vi "SetTest.vi"(0 "reference in":refnum<class "MES_Local.lvclass">, 5 "Value":variant, 11 "error in (no error)":errorcluster) -> (4 "reference in":refnum<class "MES_Local.lvclass">, 6 "Cluster 2":T1={"Code"="", "Name"="", "Description"="", "Group"="", "IsGroup"=FALSE, "Tag"="", "Method"="", "Parrameter"="", "DataType"=enum."String", "Value"=variant, "Status"=enum."Pass", "LimitLo"=variant, "LimitHi"=variant, "StringMatch"="", "BooleanMatch"=FALSE, "DisplayFormat"="", "Units"="", "TestTime"=0.0}, 8 "Complete":bool, 10 "Pass":bool, 15 "error out":errorcluster)   [LabVIEW 2022 SP3, in "MES_Local.lvlib" / "MES_Local.lvclass"]
uses:
  MES_Local.lvclass
  Components/MES_Base.lvlibp/Controls/Test.ctl
  Components/MES_Base.lvlibp/Controls/Status.ctl
  <userlib>/_OpenG.lib/string/string.llb/Trim Whitespace (String)__ogtk.vi
  <vilib>/regexp/Match Regular Expression.xnode
  Components/MES_Base.lvlibp/MES_Base.lvclass
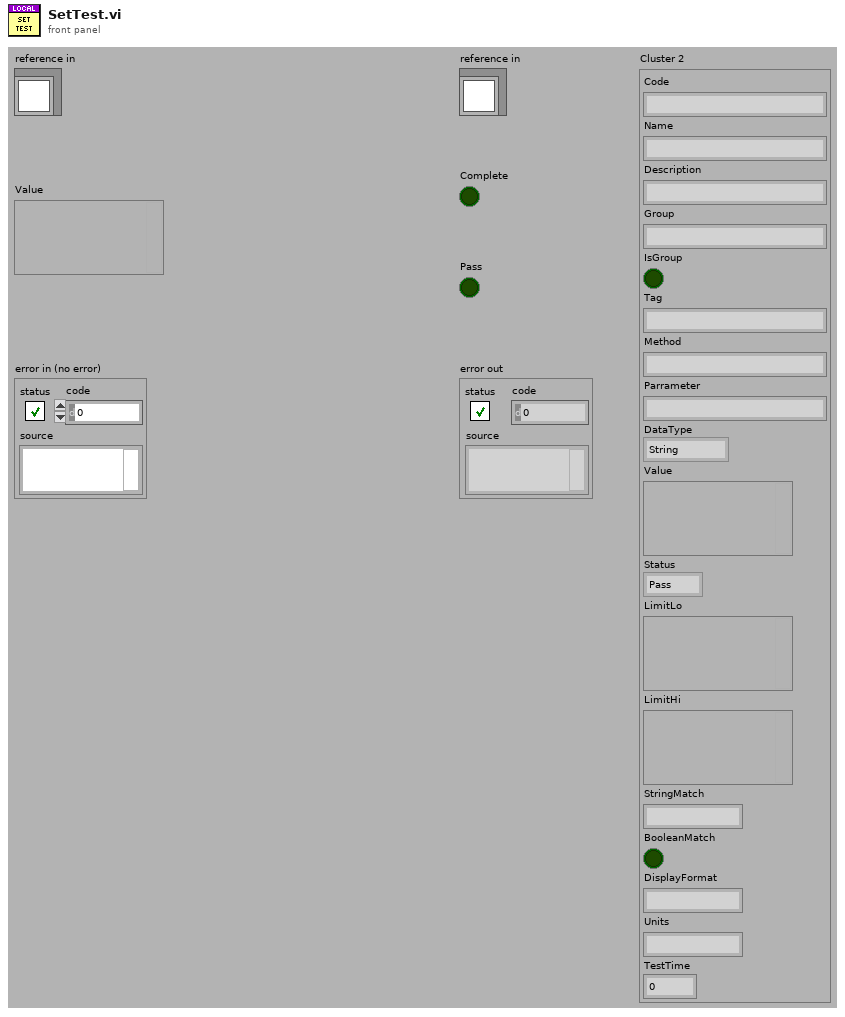
[diagram p1: front panel]
types:
  T1 = typedef "MES_Base.lvlibp/MES_Base.lvclass/Test.ctl" = cluster{"Code":string, "Name":string, "Description":string, "Group":string, "IsGroup":bool, "Tag":string, "Method":string, "Parrameter":string, "DataType":enum16{"NA", "String", "Boolean", "Int", "Dbl"}, "Value":variant, "Status":enum16{"Pending", "Pass", "Fail"}, "LimitLo":variant, "LimitHi":variant, "StringMatch":string, "BooleanMatch":bool, "DisplayFormat":string, "Units":string, "TestTime":dbl}
  T2 = typedef "MES_Base.lvlibp/MES_Base.lvclass/Status.ctl" = enum16{"Pending", "Pass", "Fail"}
  T3 = typedef "MES_Local.lvlib/MES_Local.lvclass/ObjectAttributes.ctl" = cluster{"Config":T4, "Logged_In?":bool, "AttributeNames":string[], "AttributeWritten":bool[], "ComponentNames":string[], "TestIndex":i32, "TestTag":string[], "Time Stamp":timestamp, "Employee":string, "Resource_Key":string, "Local Spec":path, "Login":refnum<class "Login_Base.lvclass">, "ReportPath":path, "Spec":T5, "StartTime":timestamp, "Role":string}
  T4 = typedef "MES_Local.lvlib/MES_Local.lvclass/Config.ctl" = cluster{"Results_Path":path}
  T5 = typedef "MES_Base.lvlibp/MES_Base.lvclass/Spec.ctl" = cluster{"Header":cluster{"Doctype":string, "Checksum":string, "DriverKey":string, "SpecId":string, "TransactionId":string, "AccountId":string, "SpecName":string, "WorkflowStep":string, "SerialNumber":string, "BatchNumber":string, "Status":enum16{"Pending", "Pass", "Fail"}, "Comment":string, "FirstFail":string, "Employee":string, "LocalMachine":string, "ResourceKey":string, "Date":string, "Time":string, "Duration":string, "DUT Position":i32}, "Components":cluster{"SerialNumber":string, "PartNumber":string, "Revision":string, "BatchNumber":string, "Name":string, "Description":string, "Attached":bool}[], "Attributes":cluster{"Name":string, "Description":string, "DataType":enum16{"NA", "String", "Boolean", "Int", "Dbl"}, "Value":variant, "DisplayFormat":string, "ReadOnly":bool, "Required":bool}[], "Tests":cluster{"Code":string, "Name":string, "Description":string, "Group":string, "IsGroup":bool, "Tag":string, "Method":string, "Parrameter":string, "DataType":enum16{"NA", "String", "Boolean", "Int", "Dbl"}, "Value":variant, "Status":enum16{"Pending", "Pass", "Fail"}, "LimitLo":variant, "LimitHi":variant, "StringMatch":string, "BooleanMatch":bool, "DisplayFormat":string, "Units":string, "TestTime":dbl}[]}
  T6 = cluster{"Code":string, "Name":string, "Description":string, "Group":string, "IsGroup":bool, "Tag":string, "Method":string, "Parrameter":string, "DataType":enum16{"NA", "String", "Boolean", "Int", "Dbl"}, "Value":variant, "Status":enum16{"Pending", "Pass", "Fail"}, "LimitLo":variant, "LimitHi":variant, "StringMatch":string, "BooleanMatch":bool, "DisplayFormat":string, "Units":string, "TestTime":dbl}[]
  T7 = cluster{"Code":string, "Name":string, "Description":string, "Group":string, "IsGroup":bool, "Tag":string, "Method":string, "Parrameter":string, "DataType":enum16{"NA", "String", "Boolean", "Int", "Dbl"}, "Value":variant, "Status":enum16{"Pending", "Pass", "Fail"}, "LimitLo":variant, "LimitHi":variant, "StringMatch":string, "BooleanMatch":bool, "DisplayFormat":string, "Units":string, "TestTime":dbl}
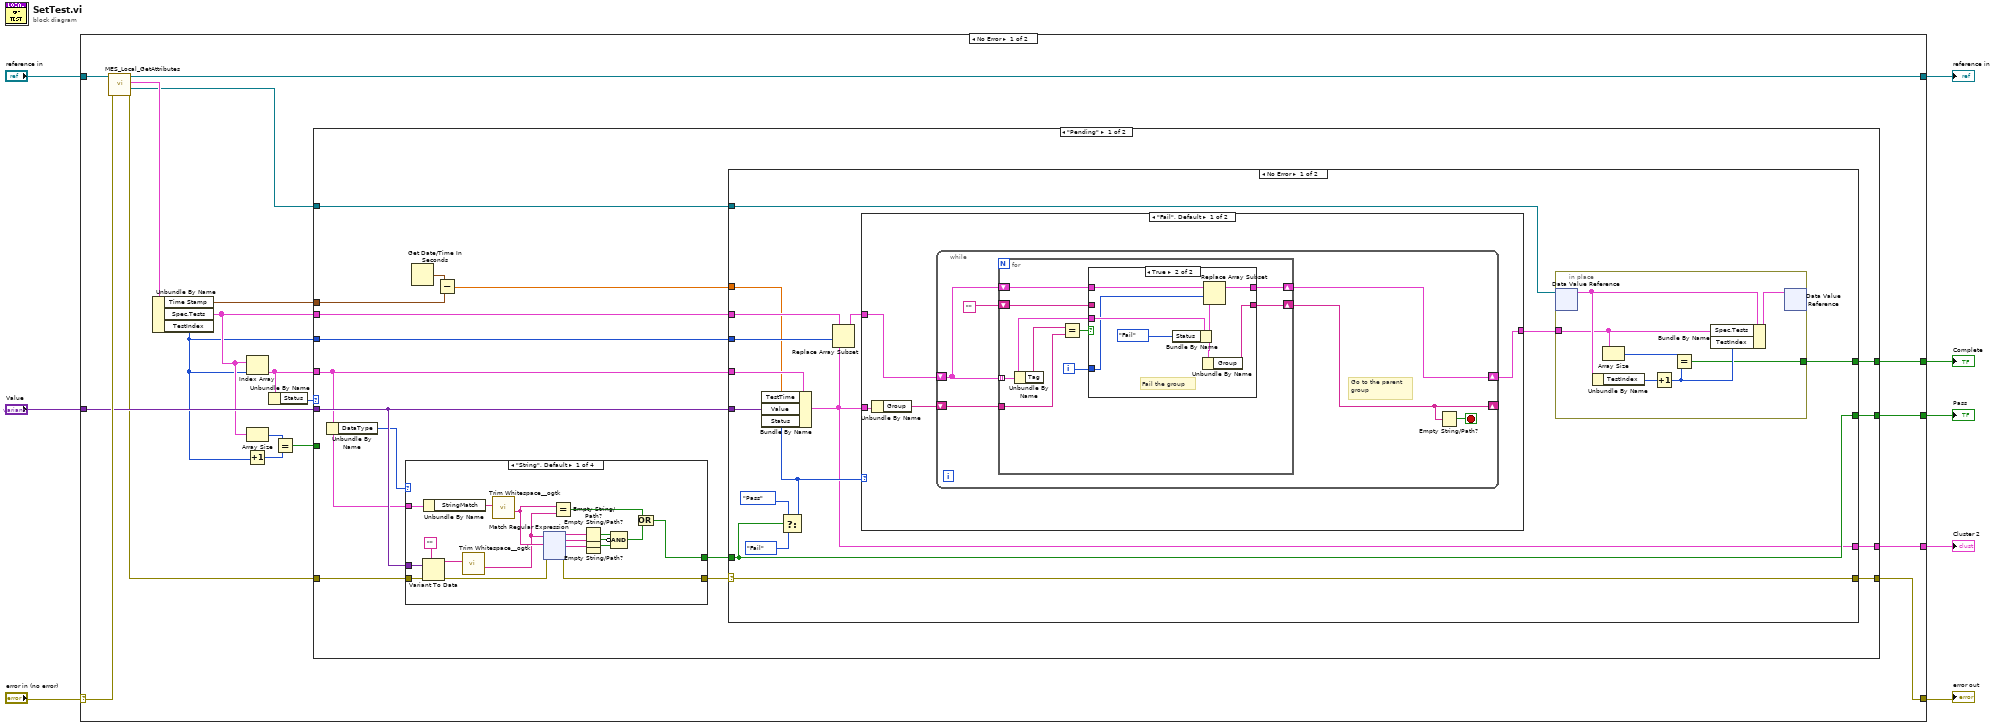
[diagram p0: block diagram]
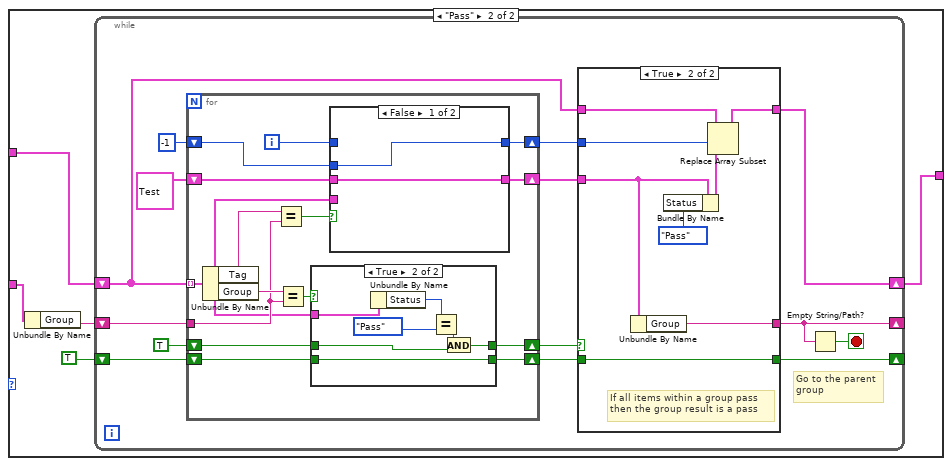
[diagram p3: hidden frame]
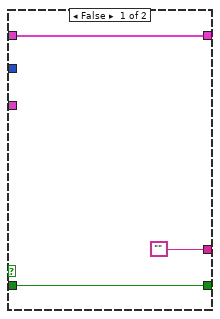
[diagram p4: hidden frame]
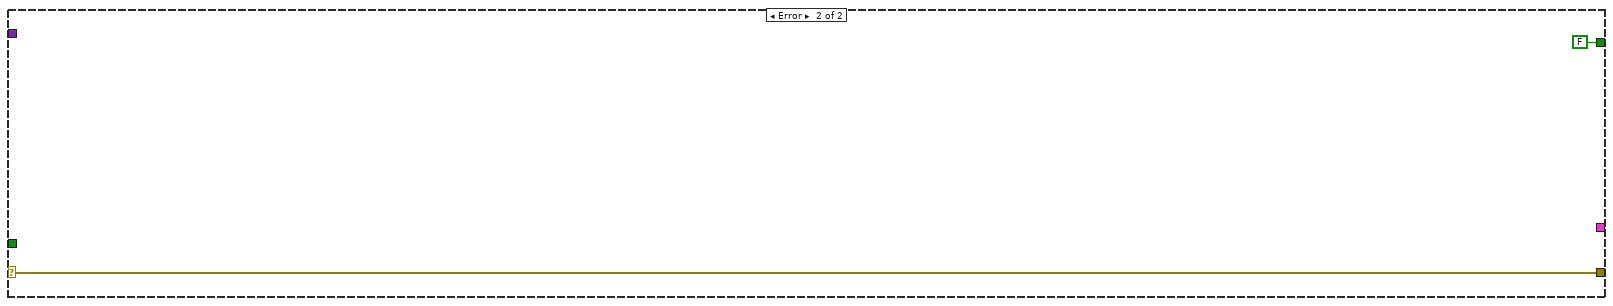
[diagram p7: hidden frame]
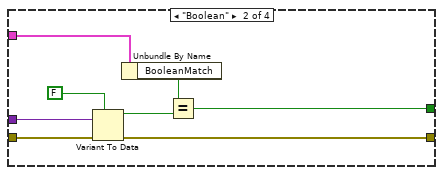
[diagram p8: hidden frame]
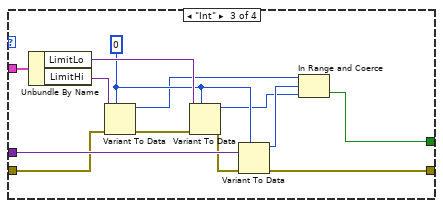
[diagram p9: hidden frame]
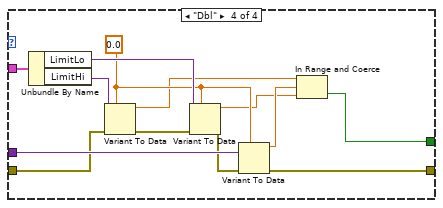
[diagram p10: hidden frame]
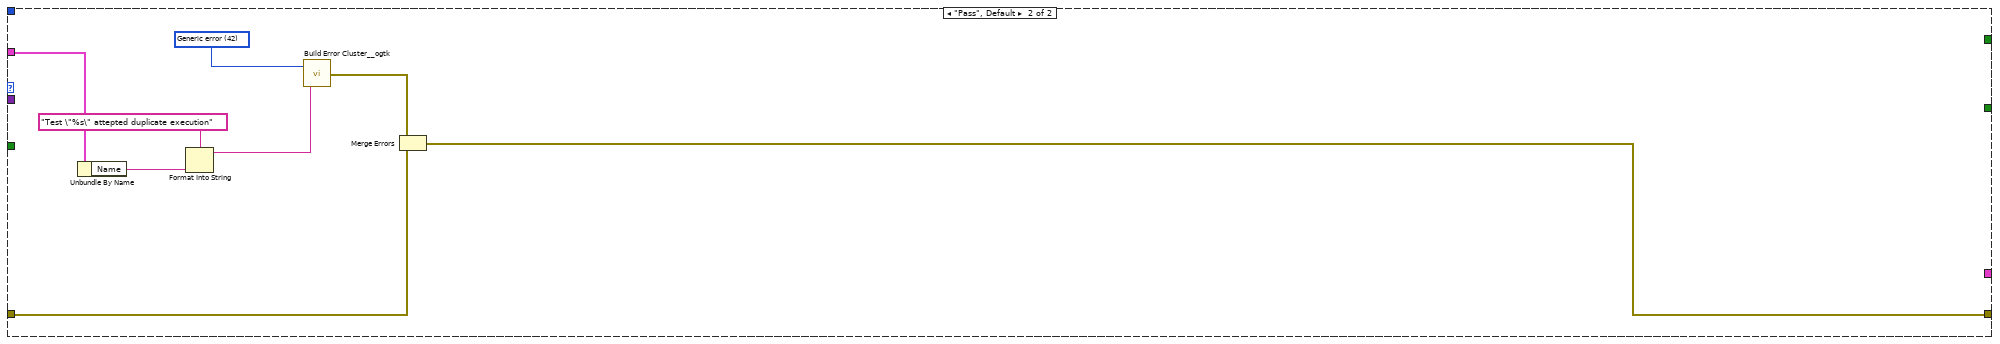
[diagram p11: hidden frame]
diagram:
  n1 = case shown="No Error" "error in (no error)" {
    selector: "error in (no error)" -> [w27 w333]
    tunnel: [w12 w333] -> w7
    tunnel: [w24 w332] -> w5
    tunnel: "reference in" -> [w25 w332]
    tunnel: "Value" -> [w19 _]
    tunnel: [w11 _] -> w3
    tunnel: [w10 _] -> w2
    tunnel: [w9 _] -> w1
    frame No Error {
      n2 = call "MES_Local_GetAttributes.vi"("error in (no error)"=w27, "reference in"=w25) -> ("error out"=w13:errorcluster, "DataRef"=w18:refnum<data-value>, "Data"=w26:T3, "reference out"=w24:refnum<class "MES_Local.lvclass">)  [unwired: 6 in]
      n3 = Unbundle By Name(w26) -> ("Time Stamp"=w17:timestamp, "Spec.Tests"=w16:T6, "TestIndex"=w15:i32)
      n4 = Index Array(array=w16, index=w15) -> (element=w23:T7)
      n5 = Increment(x=w15) -> (x+1=w20:i32)
      n6 = Array Size(array=w16) -> (size(s)=w21:i32)
      n7 = Unbundle By Name(w23) -> ("Status"=w22:enum16{"Pending", "Pass", "Fail"})
      n8 = Equal?(x=w21, y=w20) -> (x = y?=w14:bool)
      n9 = case shown="\"Pending\"" w22 {
        tunnel: w19 -> [w43 _]
        tunnel: w13 -> [w42 w329]
        tunnel: w18 -> [w41 _]
        tunnel: w16 -> [w38 _]
        tunnel: w15 -> [w37 _]
        tunnel: [w35 w328] -> w12
        tunnel: w17 -> [w33 _]
        tunnel: w23 -> [w31 w327]
        tunnel: [w30 _] -> w10
        tunnel: [w29 _] -> w9
        tunnel: [w28 _] -> w11
        tunnel: w14 -> [_ _]
        frame "Pending" {
          n10 = Unbundle By Name(w31) -> ("DataType"=w40:enum16{"NA", "String", "Boolean", "Int", "Dbl"})
          n11 = case shown="\"String\", Default" w40 {
            tunnel: w43 -> [w171 w296 w310 w323]
            tunnel: w42 -> [w172 w295 w306 w319]
            tunnel: [w161 w294 w309 w322] -> w36
            tunnel: w31 -> [w169 w293 w308 w321]
            tunnel: [w154 w290 w298 w311] -> w39
            frame "String", Default {
              n12 = Variant To Data(error in=w172, type="", Variant=w171) -> (data=w160:string, error out=w162:errorcluster)
              n13 = Unbundle By Name(w169) -> ("StringMatch"=w159:string)
              n14 = call-poly <userlib>:"Trim Whitespace__ogtk.vi"("String in"=w160) -> ("String out"=w157:string)  [unwired: 6 in]
              n15 = call-poly <userlib>:"Trim Whitespace__ogtk.vi"("String in"=w159) -> ("String out"=w158:string)  [unwired: 6 in]
              n16 = xnode "Match Regular Expression"("input string"=w157, "regular expression"=w158, "error in"=w162) -> ("before match"=w168:string, "whole match"=w165:string, "after match"=w164:string, "error out"=w161:errorcluster)  [unwired: 3 in, 1 out]
              n17 = Equal?(x=w158, y=w157) -> (x = y?=w156:bool)
              n18 = Empty String/Path?(string/path=w168) -> (empty?=w167:bool)
              n19 = Empty String/Path?(string/path=w165) -> (empty?=w166:bool)
              n20 = Empty String/Path?(string/path=w164) -> (empty?=w163:bool)
              n21 = Compound Arithmetic op=AND(w167, invert w166, w163) -> (w155:bool)
              n22 = Or(x=w156, y=w155) -> (x .or. y?=w154:bool)
            }
            frame "Boolean" {
              n23 = Variant To Data(error in=w295, type=FALSE, Variant=w296) -> (data=w292:bool, error out=w294:errorcluster)
              n24 = Unbundle By Name(w293) -> ("BooleanMatch"=w291:bool)
              n25 = Equal?(x=w291, y=w292) -> (x = y?=w290:bool)
            }
            frame "Int" {
              w302 = 0
              n26 = Unbundle By Name(w308) -> ("LimitLo"=w303:variant, "LimitHi"=w307:variant)
              n27 = Variant To Data(error in=w306, type=w302, Variant=w307) -> (data=w299:i32, error out=w305:errorcluster)
              n28 = Variant To Data(error in=w305, type=w302, Variant=w303) -> (data=w300:i32, error out=w304:errorcluster)
              n29 = Variant To Data(error in=w304, type=w302, Variant=w310) -> (data=w301:i32, error out=w309:errorcluster)
              n30 = In Range and Coerce(upper limit=w299, x=w301, lower limit=w300) -> (In Range?=w298:bool)  [unwired: 1 out]
            }
            frame "Dbl" {
              w315 = 0.0
              n31 = Unbundle By Name(w321) -> ("LimitLo"=w316:variant, "LimitHi"=w320:variant)
              n32 = Variant To Data(error in=w319, type=w315, Variant=w320) -> (data=w312:dbl, error out=w318:errorcluster)
              n33 = Variant To Data(error in=w318, type=w315, Variant=w316) -> (data=w313:dbl, error out=w317:errorcluster)
              n34 = Variant To Data(error in=w317, type=w315, Variant=w323) -> (data=w314:dbl, error out=w322:errorcluster)
              n35 = In Range and Coerce(upper limit=w312, x=w314, lower limit=w313) -> (In Range?=w311:bool)  [unwired: 1 out]
            }
          }
          n36 = Get Date/Time In Seconds() -> (seconds since 1Jan1904=w34:timestamp)
          n37 = Subtract(x=w34, y=w33) -> (x-y=w32:dbl)
          n38 = case shown="No Error" w36 {
            selector: w36 -> [w53 w153]
            tunnel: w43 -> [w58 _]
            tunnel: w41 -> [w57 _]
            tunnel: w31 -> [w56 _]
            tunnel: w39 -> [w47 _]
            tunnel: w38 -> [w51 _]
            tunnel: w37 -> [w52 _]
            tunnel: [w53 w153] -> w35
            tunnel: w32 -> [w49 _]
            tunnel: [w48 _] -> w30
            tunnel: [w47 FALSE] -> w29
            tunnel: [w46 _] -> w28
            frame No Error {
              n39 = Select(t=Status."Pass" ("Status"), s=w47, f=Status."Fail" ("Status")) -> (s? t:f=w55:T2)
              n40 = Bundle By Name(cluster=w56, "TestTime"=w49, "Value"=w58, "Status"=w55) -> (w46:T7)
              n41 = Replace Array Subset(array=w51, new element=w46, index=w52) -> (w50:T6)
              n42 = case shown="\"Fail\", Default" w55 {
                tunnel: w46 -> [w61 w91]
                tunnel: w50 -> [w62 w90]
                tunnel: [w59 w87] -> w54
                frame "Fail", Default {
                  n43 = Unbundle By Name(w61) -> ("Group"=w60:string)
                  n44 = while {
                    shift-right: [w63] -> _
                    shift-left: w60 -> [w68]
                    shift-right: [w65] -> w59
                    shift-left: w62 -> [w66]
                    stop <- w67 stop-if-true
                    # "Go to the parent\ngroup"
                    n45 = for {
                      tunnel: w68 -> [w77]
                      tunnel: w66 -> [w74] mode=indexing
                      shift-right: [w73] -> w65
                      shift-left: w66 -> [w72]
                      shift-right: [w70] -> w63
                      shift-left: "" -> [w69]
                      i -> [w71]
                      n46 = Unbundle By Name(w74) -> ("Tag"=w76:string)
                      n47 = Equal?(x=w76, y=w77) -> (x = y?=w75:bool)
                      n48 = case shown="True" w75 {
                        tunnel: w74 -> [_ w86]
                        tunnel: [w79 w84] -> w73
                        tunnel: w72 -> [w79 w85]
                        tunnel: w71 -> [_ w83]
                        tunnel: [w78 w81] -> w70
                        tunnel: w69 -> [w78 _]
                        frame False {
                        }
                        frame True {
                          # "Fail the group"
                          n49 = Bundle By Name(cluster=w86, "Status"=Status."Fail") -> (w82:T7)
                          n50 = Unbundle By Name(w82) -> ("Group"=w81:string)
                          n51 = Replace Array Subset(array=w85, new element=w82, index=w83) -> (w84:T6)
                        }
                      }
                    }
                    n52 = Empty String/Path?(string/path=w63) -> (empty?=w67:bool)
                  }
                }
                frame "Pass" {
                  n53 = Unbundle By Name(w91) -> ("Group"=w89:string)
                  n54 = while {
                    shift-right: [w104] -> _
                    shift-left: TRUE -> [w105]
                    shift-right: [w95] -> _
                    shift-left: w89 -> [w101]
                    shift-right: [w96] -> w87
                    shift-left: w90 -> [w99]
                    stop <- w93 stop-if-true
                    # "Go to the parent\ngroup"
                    n55 = for {
                      tunnel: w101 -> [w125]
                      tunnel: w99 -> [w122] mode=indexing
                      shift-right: [w128] -> w102
                      shift-left: w105 -> [w129]
                      shift-right: [w126] -> w94
                      shift-left: TRUE -> [w127]
                      shift-right: [w121] -> w100
                      shift-left: T1 {"Code"="", "Name"="", "Description"="", "Group"="", "IsGroup"=FALSE, "Tag"="", "Method"="", "Parrameter"="", "DataType"=enum."String", "Value"=variant, "Status"=enum."Pass", "LimitLo"=variant, "LimitHi"=variant, "StringMatch"="", "BooleanMatch"=FALSE, "DisplayFormat"="", "Units"="", "TestTime"=0.0} ("Cluster 2") -> [w120]
                      shift-right: [w118] -> w97
                      shift-left: -1 -> [w117]
                      i -> [w119]
                      n56 = Unbundle By Name(w122) -> ("Tag"=w124:string, "Group"=w131:string)
                      n57 = Equal?(x=w124, y=w125) -> (x = y?=w123:bool)
                      n58 = Equal?(x=w131, y=w125) -> (x = y?=w130:bool)
                      n59 = case shown="True" w130 {
                        tunnel: w129 -> [w136 w142]
                        tunnel: w122 -> [_ w144]
                        tunnel: [w136 w142] -> w128
                        tunnel: w127 -> [w137 w139]
                        tunnel: [w137 w140] -> w126
                        frame False {
                        }
                        frame True {
                          n60 = Unbundle By Name(w144) -> ("Status"=w143:enum16{"Pending", "Pass", "Fail"})
                          n61 = Equal?(x=w143, y=Status."Pass" ("Status")) -> (x = y?=w141:bool)
                          n62 = And(x=w141, y=w139) -> (x .and. y?=w140:bool)
                        }
                      }
                      n63 = case shown="False" w123 {
                        tunnel: w122 -> [_ w135]
                        tunnel: [w133 w135] -> w121
                        tunnel: w120 -> [w133 _]
                        tunnel: w119 -> [_ w134]
                        tunnel: [w132 w134] -> w118
                        tunnel: w117 -> [w132 _]
                        frame False {
                        }
                        frame True {
                          # "Get the parent"
                        }
                      }
                    }
                    n64 = case shown="True" w94 {
                      tunnel: w102 -> [w106 w116]
                      tunnel: [w106 w116] -> w104
                      tunnel: w100 -> [_ w114]
                      tunnel: ["" w115] -> w95
                      tunnel: w99 -> [w108 w113]
                      tunnel: w97 -> [_ w111]
                      tunnel: [w108 w110] -> w96
                      frame False {
                      }
                      frame True {
                        # "If all items within a group pass \nthen the group result is a pass"
                        n65 = Unbundle By Name(w114) -> ("Group"=w115:string)
                        n66 = Bundle By Name(cluster=w114, "Status"=Status."Pass") -> (w112:T1)
                        n67 = Replace Array Subset(array=w113, new element=w112, index=w111) -> (w110:T6)
                      }
                    }
                    n68 = Empty String/Path?(string/path=w95) -> (empty?=w93:bool)
                  }
                }
              }
              n69 = in-place {
                in-place-border: w54 -> [w148]
                in-place-border: [w145] -> w48
                n70 = in-place-dvr #1(w57) -> (w150:T3)  [unwired: 1 out]
                n71 = Unbundle By Name(w150) -> ("TestIndex"=w149:i32)
                n72 = Array Size(array=w148) -> (size(s)=w147:i32)
                n73 = Increment(x=w149) -> (x+1=w146:i32)
                n74 = Equal?(x=w147, y=w146) -> (x = y?=w145:bool)
                n75 = Bundle By Name(cluster=w150, "Spec.Tests"=w148, "TestIndex"=w146) -> (w151:T3)
                n76 = in-place-dvr #1(w151) -> ()  [unwired: 2 out]
              }
            }
            frame Error {
            }
          }
        }
        frame "Pass", Default {
          w331 = 42 items=["No error", "Argument error", "Memory is full", "Out of zone", "End of file", "File already open", "Generic file I/O error", "File not found", "File permission error", "Disk is full", "Duplicate path", "Too many files open", "System feature not enabled", "Resource file not found", "Cannot add resource", "Resource not found", "Image not found", "Image memory error", "Pen does not exist", "Config type invalid", "Config token not found", "Config parse error", "Config memory error", "Bad external code format", "Bad external code offset", "External code not present", "Null window", "Destroy window error", "Null menu", "Print aborted", "Bad print record", "Print driver error", "Windows error during printing", "Memory error during printing", "Print dialog error", "Generic print error", "Invalid device refnum", "Device not found", "Device parameter error", "Device unit error", "Cannot open device", "Device call aborted", "Generic error", "Cancelled by user", "Object ID too low", "Object ID too high", "Object not in heap", "Unknown heap", "Unknown object (invalid DefProc)", "Unknown object (DefProc not in table)", "Message out of range", "Invalid (null) method", "Unknown message", "Manager call not supported", "Bad address", "Network operation in progress", "Network operation timed out", "Connection is busy", "Network attribute not supported", "Network error", "Address in use", "System out of memory", "Connection aborted", "Connection refused", "Not connected", "Already connected", "Connection closed", "Initialization error (interapplication manager)", "Bad occurrence", "Wait on unbound occurrence handler", "Occurrence queue overflow", "Datalog type conflict", "Unused", "Unrecognized type (interapplication manager)", "Memory corrupt", "Failed to make temporary DLL", "Old CIN version", "Drag socket not found", "Failed to load drop-object", "Failed to register OLE object", "Failed to release OLE object", "Format specifier type mismatch", "Unknown format specifier", "Too few format specifiers", "Too many format specifiers", "Scan failed", "Newer CIN version", "Error converting to variant", "Runtime menu error", "Password tampered", "Variant attribute not found", "Incompatible variant data type", "Event data is not available", "Event Store is not present", "Occurrence is not found", "Event Queue is not created", "Event info is not available", "Refnum passed is NULL", "Error retrieving Class GUID", "Error retrieving CoClass GUID", "Error retrieving TypeLib GUID.", "Bad built application magic bytes.", "Specific driver is different from the specific driver associated with the Logical Name.", "There is no session opened to the class driver.", "Max Error", "MAX - Error with config objects", "MAX - Error loading configuration", "MAX - Group not supported"]
          n77 = Unbundle By Name(w327) -> ("Name"=w326:string)
          n78 = Format Into String(format string="Test \"%s\" attepted duplicate execution", w326) -> (resulting string=w324:string)  [unwired: 2 in, 1 out]
          n79 = call <userlib>:"Build Error Cluster__ogtk.vi"("String to Prepend to source (\"\")"=w324, "code"=w331) -> ("error out"=w330:errorcluster)
          n80 = Merge Errors(w330, w329) -> (w328:errorcluster)
        }
      }
    }
    frame Error {
    }
  }
  "error out" <- w7
  "reference in" <- w5
  "Cluster 2" <- w3
  "Complete" <- w2
  "Pass" <- w1
